vi "Set CANopen.vi"(10 "CANopen":refnum<class "CANopen.lvclass">, 11 "CANopen Actor in":refnum<class "CANopen Actor.lvclass">) -> (3 "CANopen Actor out":refnum<class "CANopen Actor.lvclass">)   [LabVIEW 2024, in "CANopen Actor.lvlib" / "CANopen Actor.lvclass"]
uses:
  CANopen Actor.lvclass
  CANopen/CANopen.lvclass
  CANopen Actor.lvclass/CANopen Actor.ctl
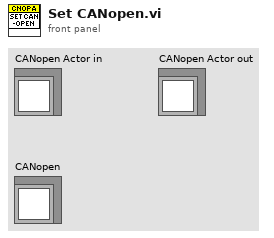
[diagram p1: front panel]
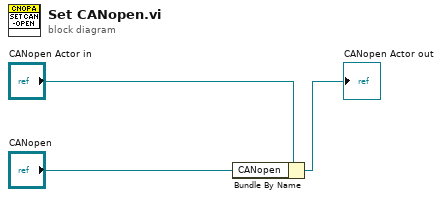
[diagram p0: block diagram]
diagram:
  n1 = Bundle By Name(cluster="CANopen Actor in", "CANopen"="CANopen") -> (→"CANopen Actor out":refnum<class "CANopen Actor.lvclass">)
